vi "In_S7F23.vi"(8 "error in (no error)":errorcluster, 11 "S7 Message Class in":refnum<class "S7 Message Class.lvclass">) -> (0 "error out":errorcluster, 1 "OK?":bool, 2 "S7F23":T1, 3 "S7 Message Class out":refnum<class "S7 Message Class.lvclass">)   [LabVIEW 2020, in "SECS Communication.lvlib" / "S7 Message Class.lvclass"]
uses:
  S7 Message Class.lvclass
  S7F23.ctl
  SECS-II Class/Format Code.ctl
  SECS-II Class/SECS-II Class.lvclass/SECS-II Class.ctl
  SECS-II Class/Variant To Data_ASCII.vi
  SECS-II Class/SECS-II Class.lvclass
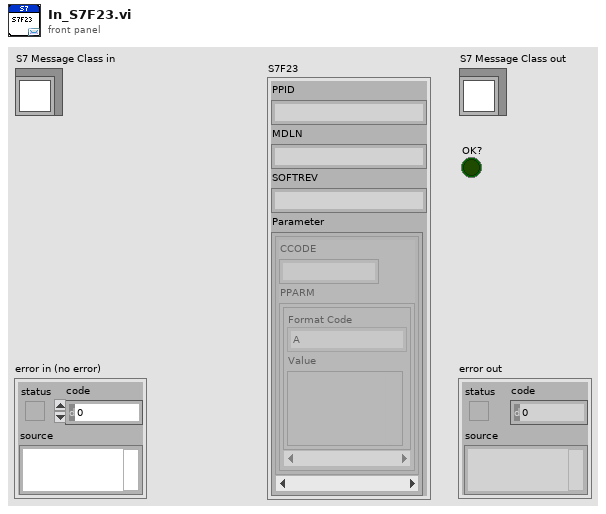
[diagram p1: front panel]
types:
  T1 = typedef "SECS Communication.lvlib/S7 Message Class.lvclass/S7F23.ctl" = cluster{"PPID":string, "MDLN":string, "SOFTREV":string, "Parameter":cluster{"CCODE":string, "PPARM":cluster{"Format Code":T2, "Value":variant}[]}[]}
  T2 = typedef "SECS Communication.lvlib/SECS-II Class.lvclass/Format Code.ctl" = enum16{"L", "A", "B", "Boolean", "J", "I1", "I2", "I4", "I8", "U1", "U2", "U4", "U8", "F4", "F8", "Char"}
  T3 = typedef "SECS Communication.lvlib/SECS-II Class.lvclass/Message Data.ctl" = cluster{"Index":i32, "Data Item Format":T4, "Format Code":T2, "Parent Index":i32, "Child Index":i32[], "Data":variant}
  T4 = typedef "SECS Communication.lvlib/SECS-II Class.lvclass/Data Item Format.ctl" = enum16{"Data Type", "Value"}
  T5 = cluster{"Data":string, cluster{"Format Code":T2, "Data":variant}[]}
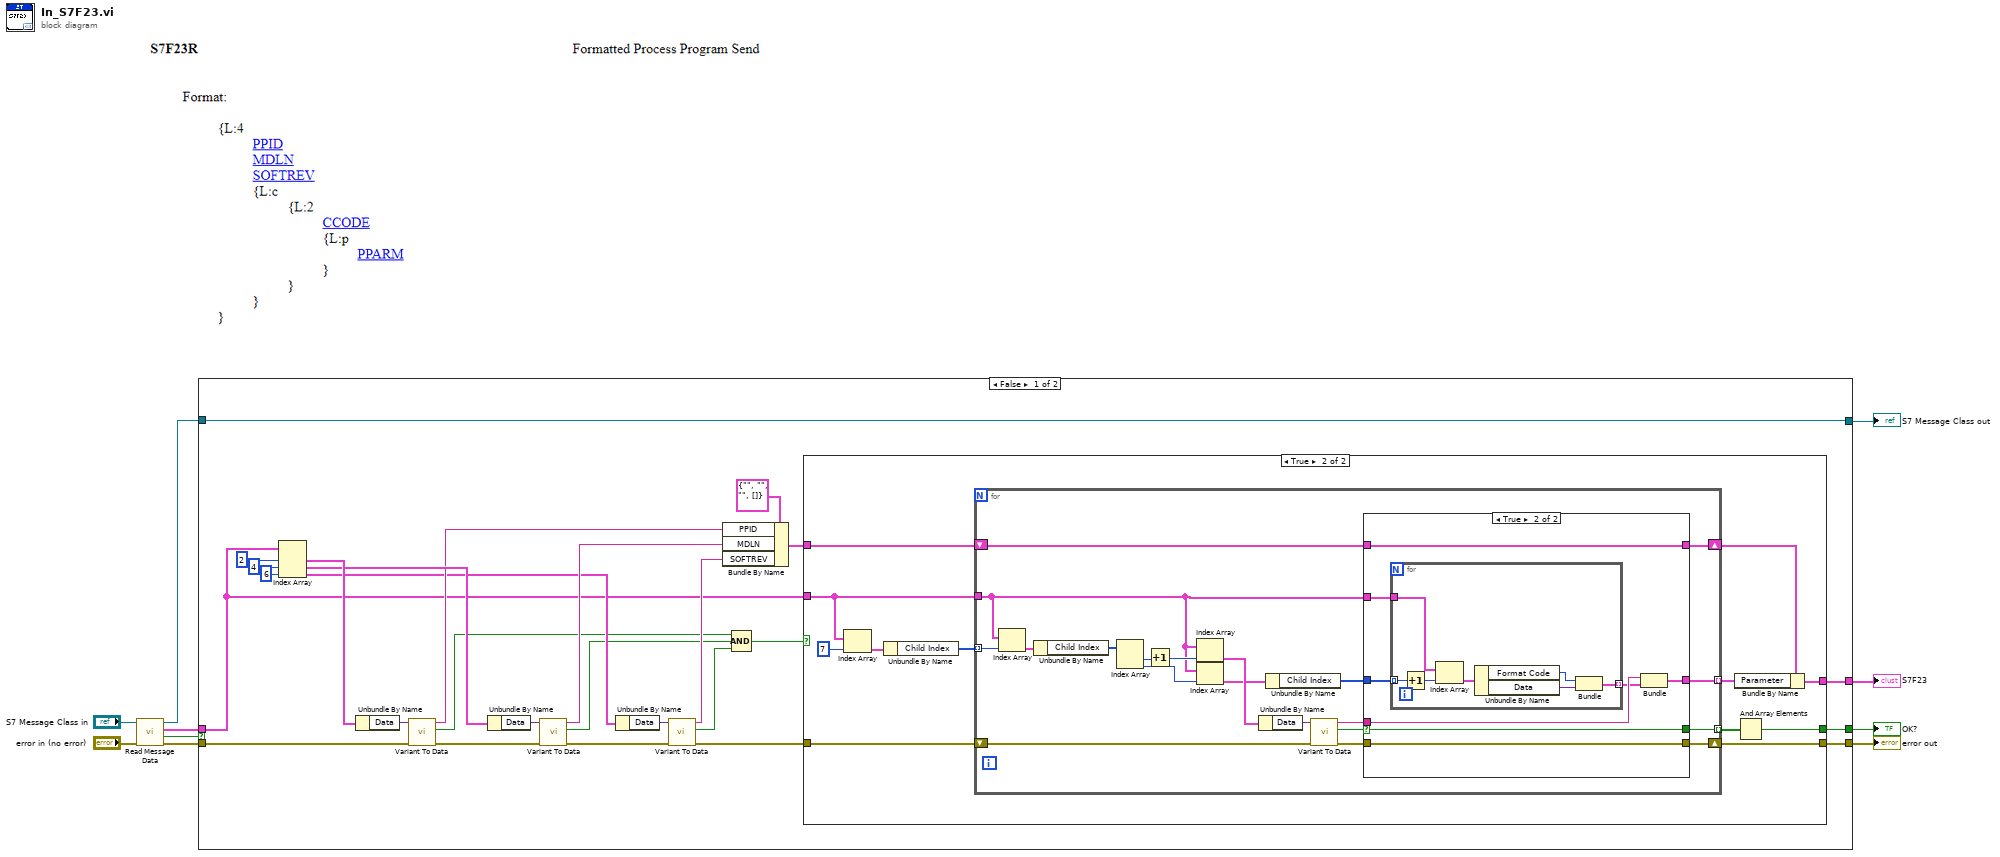
[diagram p0: block diagram]
diagram:
  n1 = call "Read Message Data.vi"("error in (no error)"="error in (no error)", "SECS-II Class in"="S7 Message Class in") -> ("error out"=w10:errorcluster, "Empty?"=w4:bool, "Message Data"=w9:T3[], "SECS-II Class out"=w2:refnum<class "S7 Message Class.lvclass">)  [unwired: 6 in]
  n2 = case shown="False" w4 {
    tunnel: w10 -> [w36 w89]
    tunnel: w9 -> [w20 _]
    tunnel: [w18 _] -> w8
    tunnel: [w17 w89] -> w7
    tunnel: [w12 _] -> w3
    tunnel: w2 -> [w11 w90]
    tunnel: [w11 w90] -> w1
    frame False {
      n3 = Index Array(array=w20, index #1=2 ("index"), index #2=4 ("index"), index #3=6 ("index")) -> (element #1=w35:T3, element #2=w30:T3, element #3=w23:T3)
      n4 = Unbundle By Name(w35) -> ("Data"=w34:variant)
      n5 = call-poly "Variant To Data.vi"("error in (no error)"=w36, "Variant"=w34) -> ("error out"=w31:errorcluster, "OK?"=w16:bool, "Data"=w28:string)  [unwired: 7 in]
      n6 = Unbundle By Name(w30) -> ("Data"=w32:variant)
      n7 = call-poly "Variant To Data.vi"("error in (no error)"=w31, "Variant"=w32) -> ("error out"=w25:errorcluster, "OK?"=w15:bool, "Data"=w27:string)  [unwired: 7 in]
      n8 = Unbundle By Name(w23) -> ("Data"=w26:variant)
      n9 = call-poly "Variant To Data.vi"("error in (no error)"=w25, "Variant"=w26) -> ("error out"=w19:errorcluster, "OK?"=w14:bool, "Data"=w22:string)  [unwired: 7 in]
      n10 = Bundle By Name(cluster=T1 {"PPID"="", "MDLN"="", "SOFTREV"="", "Parameter"=[]} ("S7F23"), "PPID"=w28, "MDLN"=w27, "SOFTREV"=w22) -> (w21:T1)
      n11 = Compound Arithmetic op=AND(w16, w15, w14) -> (w13:bool)
      n12 = case shown="True" w13 {
        tunnel: w21 -> [_ w48]
        tunnel: w20 -> [_ w46]
        tunnel: w19 -> [w38 w45]
        tunnel: [_ w43] -> w18
        tunnel: [w38 w41] -> w17
        tunnel: [_ w39] -> w12
        frame False {
        }
        frame True {
          n13 = Index Array(array=w46, index=7) -> (element=w49:T3)
          n14 = Unbundle By Name(w49) -> ("Child Index"=w47:i32[])
          n15 = for {
            shift-right: [w52] -> w44
            shift-left: w48 -> [w53]
            tunnel: w47 -> [w70] mode=indexing
            tunnel: w46 -> [w59]
            shift-right: [w54] -> w41
            shift-left: w45 -> [w68]
            tunnel: [w57] -> w42 mode=indexing
            tunnel: [w51] -> w40 mode=indexing
            n16 = Index Array(array=w59, index=w70) -> (element=w69:T3)
            n17 = Unbundle By Name(w69) -> ("Child Index"=w64:i32[])
            n18 = Index Array(array=w64) -> (element #1=w63:i32, element #2=w62:i32)  [unwired: 2 in]
            n19 = Increment(x=w63) -> (x+1=w66:i32)
            n20 = Index Array(array=w59, index=w66) -> (element=w65:T3)
            n21 = Index Array(array=w59, index=w62) -> (element=w61:T3)
            n22 = Unbundle By Name(w65) -> ("Data"=w67:variant)
            n23 = Unbundle By Name(w61) -> ("Child Index"=w60:i32[])
            n24 = call-poly "Variant To Data.vi"("error in (no error)"=w68, "Variant"=w67) -> ("error out"=w55:errorcluster, "OK?"=w56:bool, "Data"=w58:string)  [unwired: 7 in]
            n25 = case shown="True" w56 {
              selector: w56 -> [w73 w74]
              tunnel: w60 -> [_ w81]
              tunnel: w59 -> [_ w80]
              tunnel: w58 -> [_ w79]
              tunnel: [_ w77] -> w57
              tunnel: w55 -> [w72 w76]
              tunnel: [w72 w76] -> w54
              tunnel: w53 -> [w71 w75]
              tunnel: [w71 w75] -> w52
              tunnel: [w73 w74] -> w51
              frame False {
              }
              frame True {
                n26 = for {
                  tunnel: w81 -> [w83] mode=indexing
                  tunnel: w80 -> [w88]
                  tunnel: [w84] -> w78 mode=indexing
                  n27 = Increment(x=w83) -> (x+1=w82:i32)
                  n28 = Index Array(array=w88, index=w82) -> (element=w87:T3)
                  n29 = Unbundle By Name(w87) -> ("Format Code"=w85:T2, "Data"=w86:variant)
                  n30 = Bundle("Format Code"=w85, "Data"=w86) -> (w84:cluster{"Format Code":T2, "Data":variant})  [unwired: 1 in]
                }
                n31 = Bundle("Data"=w79, w78) -> (w77:T5)  [unwired: 1 in]
              }
            }
          }
          n32 = Bundle By Name(cluster=w44, "Parameter"=w42) -> (w43:T1)
          n33 = And Array Elements(Boolean array=w40) -> (logical AND=w39:bool)
        }
      }
    }
    frame True {
    }
  }
  "error out" <- w7
  "S7 Message Class out" <- w1
  "S7F23" <- w8
  "OK?" <- w3
